vi "Sort Triangles.vi"(11 "Triangles":T3[](array[typedef])) -> (3 "Triangles Sorted":T1[](array[typedef]))   [LabVIEW 2020, in "3D.lvlib"]
uses:
  3D.lvlib
  Triangle 3D.ctl
  Vector 3D.ctl
  Triangle 2D.ctl
  Point 2D.ctl
  <userlib>/_OpenG.lib/array/array.llb/Sort 1D Array (SGL)__ogtk.vi
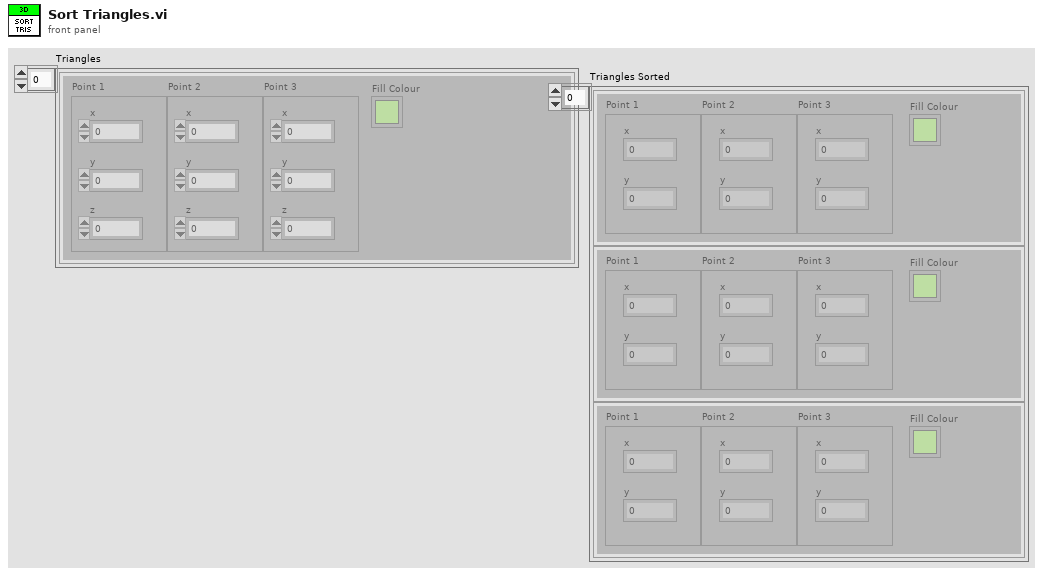
[diagram p1: front panel]
types:
  T1 = typedef "3D.lvlib/Triangle 2D.ctl" = cluster{"Point 1":T2, "Point 2":T2, "Point 3":T2, "Fill Colour":u32}
  T2 = typedef "3D.lvlib/Point 2D.ctl" = cluster{"x":sgl, "y":sgl}
  T3 = typedef "3D.lvlib/Triangle 3D.ctl" = cluster{"Point 1":T4, "Point 2":T4, "Point 3":T4, "Fill Colour":u32}
  T4 = typedef "3D.lvlib/Vector 3D.ctl" = cluster{"x":sgl, "y":sgl, "z":sgl}
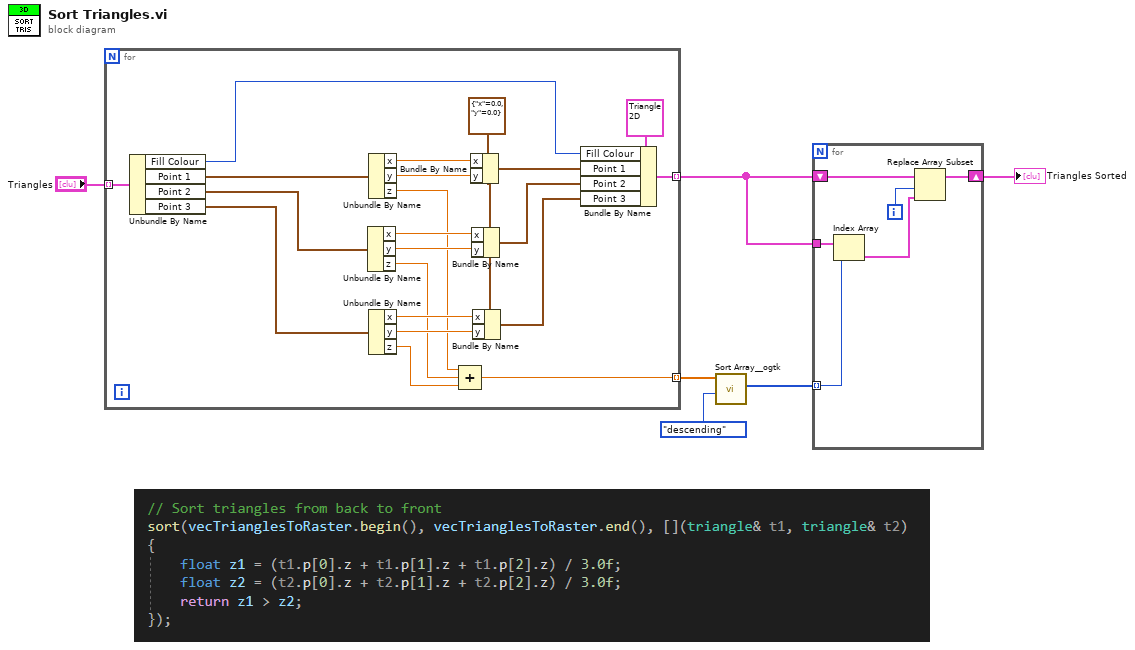
[diagram p0: block diagram]
diagram:
  n1 = for {
    tunnel: "Triangles" -> [w26] mode=indexing
    tunnel: [w25] -> w3 mode=indexing
    tunnel: [w8] -> w5 mode=indexing
    w23 = T2 {"x"=0.0, "y"=0.0} ("Point 1")
    n2 = Unbundle By Name(w26) -> ("Fill Colour"=w7:u32, "Point 1"=w14:T4, "Point 2"=w13:T4, "Point 3"=w12:T4)
    n3 = Unbundle By Name(w13) -> ("x"=w18:sgl, "y"=w17:sgl, "z"=w10:sgl)
    n4 = Unbundle By Name(w14) -> ("x"=w20:sgl, "y"=w19:sgl, "z"=w11:sgl)
    n5 = Unbundle By Name(w12) -> ("x"=w16:sgl, "y"=w15:sgl, "z"=w9:sgl)
    n6 = Compound Arithmetic op=ADD(w11, w10, w9) -> (w8:sgl)
    n7 = Bundle By Name(cluster=w23, "x"=w20, "y"=w19) -> (w24:T2)
    n8 = Bundle By Name(cluster=w23, "x"=w18, "y"=w17) -> (w22:T2)
    n9 = Bundle By Name(cluster=w23, "x"=w16, "y"=w15) -> (w21:T2)
    n10 = Bundle By Name(cluster=T1 {"Point 1"={"x"=0.0, "y"=0.0}, "Point 2"={"x"=0.0, "y"=0.0}, "Point 3"={"x"=0.0, "y"=0.0}, "Fill Colour"=12517256} ("Triangle 2D"), "Fill Colour"=w7, "Point 1"=w24, "Point 2"=w22, "Point 3"=w21) -> (w25:T1)
  }
  n11 = call-poly <userlib>:"Sort Array__ogtk.vi"("Order"=enum16{"ascending", "descending"}."descending", "Array in"=w5) -> ("Sorted Pointers"=w4:i32[])  [unwired: 8 in, 1 out]
  n12 = for {
    tunnel: w4 -> [w31] mode=indexing
    tunnel: w3 -> [w32]
    shift-right: [w29] -> w2
    shift-left: w3 -> [w30]
    i -> [w33]
    n13 = Index Array(array=w32, index=w31) -> (element=w28:T1)
    n14 = Replace Array Subset(array=w30, new element=w28, index=w33) -> (w29:T1[])
  }
  "Triangles Sorted" <- w2
